vi "Stop Triggered Log.vi"(8 "error in (no error)":errorcluster, 11 "Triggered Log in":refnum<class "Triggered Log.lvclass">) -> (0 "error out":errorcluster, 3 "Segmented Log Ref":refnum<data-value>)   [LabVIEW 2015, in "Triggered Log.lvclass"]
doc: "This VI stops the triggered log. It flushes any remaning data in the data buffer to disk and finalizes the start and stop triggers. It returns the segmented log reference that was passed to the triggered log when it was created. It does not stop or finalize the segmented log."
uses:
  Triggered Log.lvclass
  Engine/Classes/Logs/Segmented Logs/Segmented Log/Segmented Log.lvclass
  Triggered Log State.ctl
  Triggered Log.lvclass/Triggered Log.ctl
  Engine/Classes/Logs/Segmented Logs/Segmented Log/Segmented Log.lvclass/Segmented Log.ctl
  Shared/Classes/Log File Specifications/Log File Specification/Log File Specification.lvclass/Log File Specification.ctl
  Engine/Classes/Logs/Segmented Logs/Footprint Segmented Log/Footprint Segmented Log.lvclass/Footprint Segmented Log.ctl
  Engine/Classes/Logs/Log Files/Log File/Log File.lvclass/Log File.ctl
  Engine/Classes/Logs/Segmented Logs/Time Segmented Log/Time Segmented Log.lvclass/Time Segmented Log.ctl
  Engine/Classes/Logs/Log Files/TDMS Log File/TDMS Log File.lvclass/TDMS Log File.ctl
  Engine/Classes/Logs/Log Files/Text Log File/Text Log File.lvclass/Text Log File.ctl
  Flush Buffer Data to File.vi
  On Triggered Log State Change.vi
  Engine/Classes/Triggers/Trigger/Initialize.vi
  Flush Buffer Data.vi
  Engine/Classes/Logs/Segmented Logs/Segmented Log/Write Data to Log File Instance (Waveform).vi
  Engine/Classes/Logs/Segmented Logs/Segmented Log/Write Data to Log File Instance.vi
  Engine/Classes/Triggers/Digital Edge Trigger/Initialize Digital Edge Trigger.vi
  Engine/Classes/Triggers/Analog Edge Trigger/Initialize Analog Edge Trigger.vi
  Engine/Classes/Triggers/Value Change Trigger/Initialize Value Change Trigger.vi
  Engine/Classes/Logs/Segmented Logs/Segmented Log/Check Close File.vi
  Engine/Classes/Logs/Segmented Logs/Segmented Log/Check Open File.vi
  Engine/Classes/Logs/Segmented Logs/Segmented Log/Close Log File Instance.vi
  Engine/Classes/Logs/Segmented Logs/Segmented Log/Segment Log File.vi
  Engine/Classes/Logs/Segmented Logs/Segmented Log/Open Log File Instance.vi
  Engine/Classes/Logs/Log Files/Log File/Close Log File.vi
  Engine/Classes/Logs/Segmented Logs/Segmented Log/Make File Read-Only.vi
  Engine/Classes/Logs/Segmented Logs/Segmented Log/On Segmented Log Complete.vi
  Engine/Classes/Logs/Segmented Logs/Segmented Log/On File Close.vi
  Engine/Classes/Logs/Segmented Logs/Footprint Segmented Log/Segment Log File (Footprint).vi
  Engine/Classes/Logs/Segmented Logs/Time Segmented Log/Segment Log File (Time).vi
  Shared/Classes/Log File Specifications/Log File Specification/Open Log File.vi
  Shared/Classes/Log File Specifications/Log File Specification/Set Path Tag.vi
  Engine/Classes/Logs/Segmented Logs/Segmented Log/On File Open.vi
  Shared/Classes/Log File Specifications/Log File Specification/Set Filename Offset.vi
  Engine/Classes/Logs/Log Files/TDMS Log File/Close TDMS Log File.vi
  Engine/Classes/Logs/Log Files/Text Log File/Close Text Log File.vi
  Engine/Classes/Logs/Segmented Logs/Segmented Log/Get Current Log File Instance.vi
  Engine/Classes/Logs/Log Files/Log File/Get File Size.vi
  Engine/Classes/Logs/Log Files/Log File/Get Start Time.vi
  Shared/Classes/Log File Specifications/Log File Specification/Build File Path.vi
  Shared/Classes/Log File Specifications/Log File Specification/Resolve File Conflicts.vi
  Engine/Classes/Triggers/Trigger/Finalize.vi
  Engine/Classes/Logs/Log Files/Log File/Write to Log File.vi
  <vilib>/Utility/error.llb/Error Cluster From Error Code.vi
  Shared/Classes/Log File Specifications/Log File Specification/Initialize Log File.vi
  <vilib>/Utility/libraryn.llb/Create Directory Recursive.vi
  <vilib>/Utility/libraryn.llb/Check if File or Folder Exists.vi
  <vilib>/Utility/libraryn.llb/Get File Extension.vi
  Engine/Classes/Logs/Log Files/Log File/Write to Log File (Waveform).vi
  Engine/Classes/Triggers/Value Change Trigger/Value Change Trigger.lvclass
  Engine/Classes/Triggers/Analog Edge Trigger/Analog Edge Trigger.lvclass
  Engine/Classes/Triggers/Digital Edge Trigger/Digital Edge Trigger.lvclass
  Engine/Classes/Logs/Log Files/Text Log File/Text Log File.lvclass
  Engine/Classes/Logs/Log Files/TDMS Log File/TDMS Log File.lvclass
  Engine/Classes/Logs/Log Files/Log File/Log File.lvclass
  Engine/Classes/Logs/Segmented Logs/Time Segmented Log/Time Segmented Log.lvclass
  Engine/Classes/Logs/Segmented Logs/Footprint Segmented Log/Footprint Segmented Log.lvclass
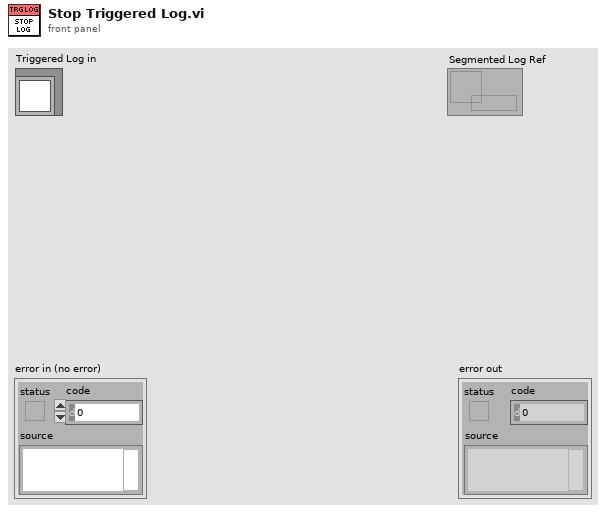
[diagram p1: front panel]
types:
  T1 = typedef "Triggered Log.lvclass/Triggered Log State.ctl" = enum16{"Waiting on Trigger", "Triggered", "Posttrigger", "Complete", "Idle", "Error"}
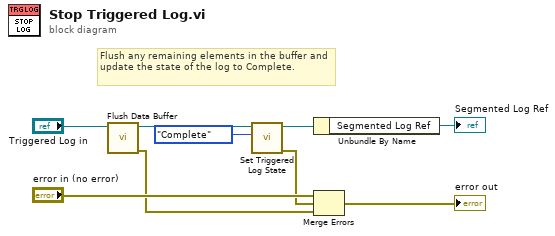
[diagram p0: block diagram]
diagram:
  # "Flush any remaining elements in the buffer and update the state of the log to Complete."
  n1 = call "Flush Data Buffer.vi"("Triggered Log in"="Triggered Log in") -> ("error out"=w5:errorcluster, "Triggered Log out"=w4:refnum<class "Triggered Log.lvclass">)  [unwired: 9 in]
  n2 = call "Set Triggered Log State.vi"("Triggered Log State"=Triggered_Log_State."Complete", "Triggered Log in"=w4) -> ("error out"=w1:errorcluster, "Triggered Log out"=w2:refnum<class "Triggered Log.lvclass">)  [unwired: 8 in]
  n3 = Unbundle By Name(w2) -> ("Segmented Log Ref"=→"Segmented Log Ref":refnum<data-value>)
  n4 = Merge Errors("error in (no error)", w1, w5) -> (→"error out":errorcluster)
